vi "Core Main.vi"(10 "Vision":T1, 11 "Referee":T2) -> ()   [LabVIEW 2016]
uses:
  <extravilib>/ChannelInstances/Lossy Stream-t'SSL Referee Game Status.ctl'/)Channel.ctl
  SSL Referee Game Status.ctl
  <extravilib>/ChannelInstances/Lossy Stream-c(t'SSL Detection Frame.ctl',c(u32,u32,u32,u32,u32,u32,u32,u32,u32,u32,u32,u32,u32,u32))/)Channel.ctl
  SSL Detection Robot.ctl
  SSL Detection Ball.ctl
  <extravilib>/ChannelInstances/Lossy Stream-a[.](t'AI Robot.ctl')/Read With Abort.vi
  <extravilib>/ChannelInstances/Lossy Stream-t'AI Input.ctl'/Read With Abort.vi
  <extravilib>/ChannelInstances/Lossy Stream-a[.](t'AI Robot.ctl')/Write With Abort.vi
  <extravilib>/ChannelInstances/Lossy Stream-t'SSL Referee Game Status.ctl'/Read With Abort.vi
  <extravilib>/ChannelInstances/Lossy Stream-c(t'SSL Detection Frame.ctl',c(u32,u32,u32,u32,u32,u32,u32,u32,u32,u32,u32,u32,u32,u32))/Read With Abort.vi
  <extravilib>/ChannelInstances/Lossy Stream-t'AI Input.ctl'/Write With Abort.vi
  <extravilib>/ChannelInstances/Lossy Stream-a[.](t'AI Robot.ctl')/Endpoint.vi
  <extravilib>/ChannelInstances/Lossy Stream-t'AI Input.ctl'/Endpoint.vi
  <extravilib>/ChannelInstances/Lossy Stream-t'SSL Referee Game Status.ctl'/Endpoint.vi
  <extravilib>/ChannelInstances/Lossy Stream-c(t'SSL Detection Frame.ctl',c(u32,u32,u32,u32,u32,u32,u32,u32,u32,u32,u32,u32,u32,u32))/Endpoint.vi
  <extravilib>/ChannelInstances/Lossy Stream-a[.](t'AI Robot.ctl')/Instantiate.vi
  <extravilib>/ChannelInstances/Lossy Stream-a[.](t'AI Robot.ctl')/)Channel.vi
  <resource>/ChannelSupport/_ChannelSupport/WaitIfNeeded.vi
  <extravilib>/ChannelInstances/Lossy Stream-t'AI Input.ctl'/Instantiate.vi
  <extravilib>/ChannelInstances/Lossy Stream-t'AI Input.ctl'/)Channel.vi
  <extravilib>/ChannelInstances/Lossy Stream-t'SSL Referee Game Status.ctl'/)Channel.vi
  <extravilib>/ChannelInstances/Lossy Stream-c(t'SSL Detection Frame.ctl',c(u32,u32,u32,u32,u32,u32,u32,u32,u32,u32,u32,u32,u32,u32))/)Channel.vi
  <extravilib>/ChannelInstances/Lossy Stream-c(t'SSL Detection Frame.ctl',c(u32,u32,u32,u32,u32,u32,u32,u32,u32,u32,u32,u32,u32,u32)).lvlib
  <extravilib>/ChannelInstances/Lossy Stream-t'SSL Referee Game Status.ctl'.lvlib
  <extravilib>/ChannelInstances/Lossy Stream-t'AI Input.ctl'.lvlib
  <extravilib>/ChannelInstances/Lossy Stream-a[.](t'AI Robot.ctl').lvlib
panel:
  # "Score"
  # "Red Cards"
  # "Yellow Cards"
  # "Timeouts Left"
  # "Timeout Remaining"
  # "Goalie ID"
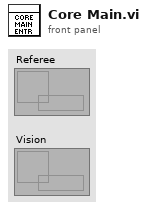
[diagram p1: front panel]
types:
  T1 = typedef "Lossy Stream-c(t'SSL Detection Frame.ctl',c(u32,u32,u32,u32,u32,u32,u32,u32,u32,u32,u32,u32,u32,u32)).lvlib/)Channel.ctl" = refnum<queue>
  T2 = typedef "Lossy Stream-t'SSL Referee Game Status.ctl'.lvlib/)Channel.ctl" = refnum<queue>
  T3 = typedef "SSL Detection Robot.ctl" = cluster{"x":dbl, "robot_id":u32, "confidence":sgl, "y":sgl, "orientation":sgl, "pixel_x":sgl, "pixel_y":sgl, "height":sgl, "Valid":bool, "Time Stamp":timestamp}
  T4 = typedef "SSL Detection Ball.ctl" = cluster{"x":sgl, "area":u32, "confidence":sgl, "y":sgl, "z":sgl, "pixel_x":sgl, "pixel_y":sgl, "Valid":bool, "Time Stamp":timestamp}
  T5 = cluster{"Detection Frame":cluster{"frame_number":u32, "t_capture":dbl, "t_sent":dbl, "camera_id":u32, "robots_yellow":T3[], "robots_blue":T3[], "balls":T4[], "Valid":bool, "Time Stamp":timestamp}, "Field Size":cluster{"line_width":u32, "field_length":u32, "field_width":u32, "boundary_width":u32, "referee_width":u32, "goal_width":u32, "goal_depth":u32, "goal_wall_width":u32, "center_circle_radius":u32, "defense_radius":u32, "defense_stretch":u32, "free_kick_from_defense_dist":u32, "penalty_spot_from_field_line_dist":u32, "penalty_line_from_spot_dist":u32}}
  T6 = typedef "SSL Referee Game Status.ctl" = cluster{"Stage":string, "Command":string, "Time Left":dbl, "Yellow Team":string, "Blue Team":string, "Yellow Score":u32, "Blue Score":u32, "Yellow Red Cards":u32, "Blue Red Cards":u32, "Yellow Yellow Cards":u32, "Blue Yellow Cards":u32, "Yellow Timeouts Left":u32, "Blue Timeouts Left":u32, "Yellow Timeout Remaining":dbl, "Blue Timeout Remaining":dbl, "Yellow Goalie Id":u32, "Blue Goalie Id":u32, "Time":timestamp}
  T7 = cluster{"frame_number":u32, "t_capture":dbl, "t_sent":dbl, "camera_id":u32, "robots_yellow":T3[], "robots_blue":T3[], "balls":T4[], "Valid":bool, "Time Stamp":timestamp}
  T8 = cluster{"line_width":u32, "field_length":u32, "field_width":u32, "boundary_width":u32, "referee_width":u32, "goal_width":u32, "goal_depth":u32, "goal_wall_width":u32, "center_circle_radius":u32, "defense_radius":u32, "defense_stretch":u32, "free_kick_from_defense_dist":u32, "penalty_spot_from_field_line_dist":u32, "penalty_line_from_spot_dist":u32}
  T9 = typedef "AI Input.ctl" = cluster{"our_robots":T10[], "enemy_robots":T10[], "balls":T11[], "geometry":T12, "IA Judge":T13}
  T10 = typedef "AI Robot.ctl" = cluster{"id":u32, "function":enum16{"Attacker", "Goalie", "Defender"}, "x":dbl, "y":dbl, "orientation":dbl, "v_x":dbl, "v_y":dbl, "v_ang":dbl, "kick_x":dbl, "kick_z":dbl, "dribble":bool, "Timestamp":timestamp}
  T11 = typedef "AI Ball.ctl" = cluster{"x":dbl, "y":dbl, "timestamp":timestamp}
  T12 = typedef "Field Size.ctl" = cluster{"line_width":u32, "field_length":u32, "field_width":u32, "boundary_width":u32, "referee_width":u32, "goal_width":u32, "goal_depth":u32, "goal_wall_width":u32, "center_circle_radius":u32, "defense_radius":u32, "defense_stretch":u32, "free_kick_from_defense_dist":u32, "penalty_spot_from_field_line_dist":u32, "penalty_line_from_spot_dist":u32}
  T13 = typedef "AI Judge.ctl" = cluster{"stage":string, "command":string, "our_goalie_id":dbl, "enemy_goalie_id":dbl}
  T14 = typedef "Lossy Stream-t'AI Input.ctl'.lvlib/)Channel.ctl" = refnum<queue>
  T15 = typedef "Lossy Stream-a[.](t'AI Robot.ctl').lvlib/)Channel.ctl" = refnum<queue>
  T16 = typedef "grSim Robot Command.ctl" = cluster{"id":u32, "kickspeedx":sgl, "kickspeedz":sgl, "veltangent":sgl, "velnormal":sgl, "velangular":sgl, "spinner":bool, "wheelspeed":bool, "wheel1":sgl, "wheel2":sgl, "wheel3":sgl, "wheel4":sgl}
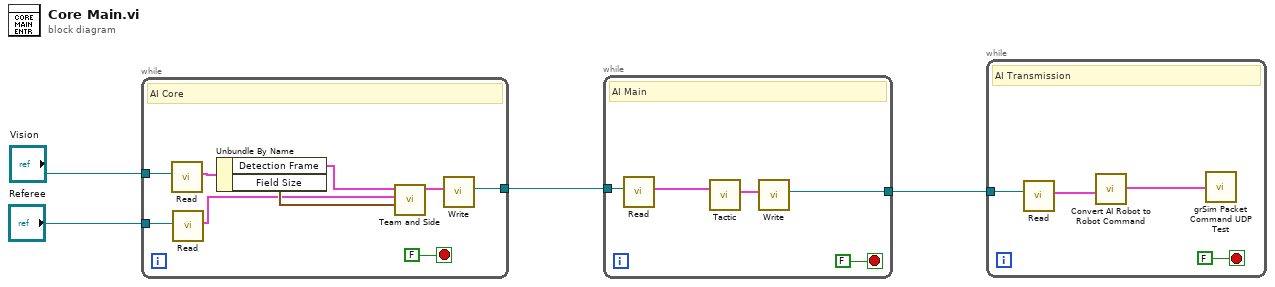
[diagram p0: block diagram]
diagram:
  n1 = while {
    tunnel: "Vision" -> [w13]
    tunnel: [w6] -> w4
    tunnel: "Referee" -> [w5]
    stop <- FALSE stop-if-true
    # "AI Core"
    n2 = call <extravilib>:"Read.vi"("channel"=w13) -> ("element"=w12:T5)  [unwired: 5 in, 5 out]
    n3 = call <extravilib>:"Read.vi"("channel"=w5) -> ("element"=w9:T6)  [unwired: 5 in, 5 out]
    n4 = Unbundle By Name(w12) -> ("Detection Frame"=w11:T7, "Field Size"=w10:T8)
    n5 = call "Team and Side.vi"("Field Size 2"=w10, "Game Status"=w9, "Input Detection Frame"=w11) -> ("Output IA Input"=w7:T9)  [unwired: 8 in]
    n6 = call <extravilib>:"Write.vi"("element"=w7) -> ("channel"=w6:T14)  [unwired: 8 in, 2 out]
  }
  n7 = while {
    tunnel: w4 -> [w18]
    tunnel: [w14] -> w1
    stop <- FALSE stop-if-true
    # "AI Main"
    n8 = call <extravilib>:"Read.vi"("channel"=w18) -> ("element"=w16:T9)  [unwired: 5 in, 5 out]
    n9 = call "Tactic.vi"("Output IA Main"=w16) -> ("Output Array"=w15:T10[])  [unwired: 10 in]
    n10 = call <extravilib>:"Write.vi"("element"=w15) -> ("channel"=w14:T15)  [unwired: 8 in, 2 out]
  }
  n11 = while {
    tunnel: w1 -> [w21]
    stop <- FALSE stop-if-true
    # "AI Transmission"
    n12 = call <extravilib>:"Read.vi"("channel"=w21) -> ("element"=w20:T10[])  [unwired: 5 in, 5 out]
    n13 = call "Convert AI Robot to Robot Command.vi"("Input Array"=w20) -> ("Output Array"=w19:T16[])
    n14 = call "grSim Packet Command UDP Test.vi"("Robots"=w19) -> ()
  }
